vi "Prime.vi"() -> ()   [LabVIEW 2012]
panel:
  out "s? t:f":string
  in  "Numeric":dbl
  out "Boolean":bool
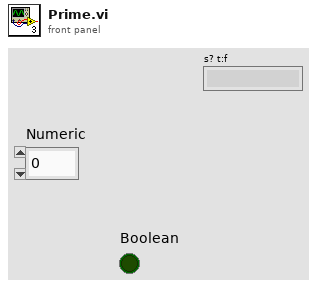
[diagram p1: front panel]
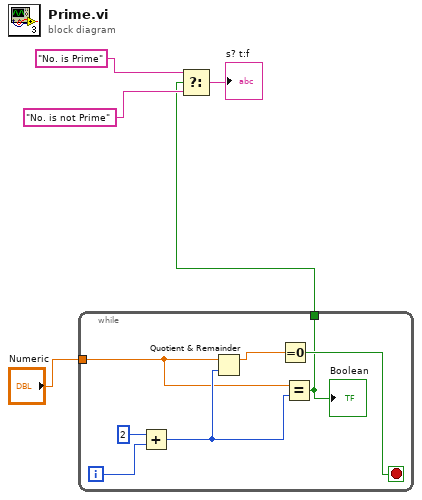
[diagram p0: block diagram]
diagram:
  n1 = while {
    tunnel: "Numeric" -> [w8]
    tunnel: [w6] -> w1
    i -> [w9]
    stop <- w7 stop-if-true
    n2 = Add(x=i16 2, y=w9) -> (x+y=w11:i32)
    n3 = Quotient & Remainder(x=w8, y=w11) -> (x-y*floor(x/y)=w12:dbl)  [unwired: 1 out]
    n4 = Equal To 0?(x=w12) -> (x = 0?=w7:bool)
    n5 = Equal?(x=w8, y=w11) -> (x = y?=w6:bool)
    "Boolean" <- w6
  }
  n6 = Select(t="No. is Prime", s=w1, f="No. is not Prime") -> (s? t:f=→"s? t:f":string)
